vi "Time calculation.vi"(0 "Time between marks (ticks)":u32, 1 "Mode":enum16{"Auto Calc Tpulse", "Auto Calc Tb"}(ring), 5 "Ta (ticks)":i32, 7 "Tb (ticks)":i32, 9 "Number of pulses (N)":i32=4, 11 "TPulse (ticks)":i32=2000) -> (4 "appended array":i32[](array[numeric]), 6 "Ta Error":bool, 8 "Tb Error":bool, 10 "Tpulse Error":bool, 15 "Remainder (ticks)":i32)   [LabVIEW 2014]
panel:
  out "Tpulse OK?":bool
  out "Tb OK?":bool
  out "Ta OK?":bool
  out "Ta Out":i32
  out "Tb Out":i32
  out "TPulse Out":i32
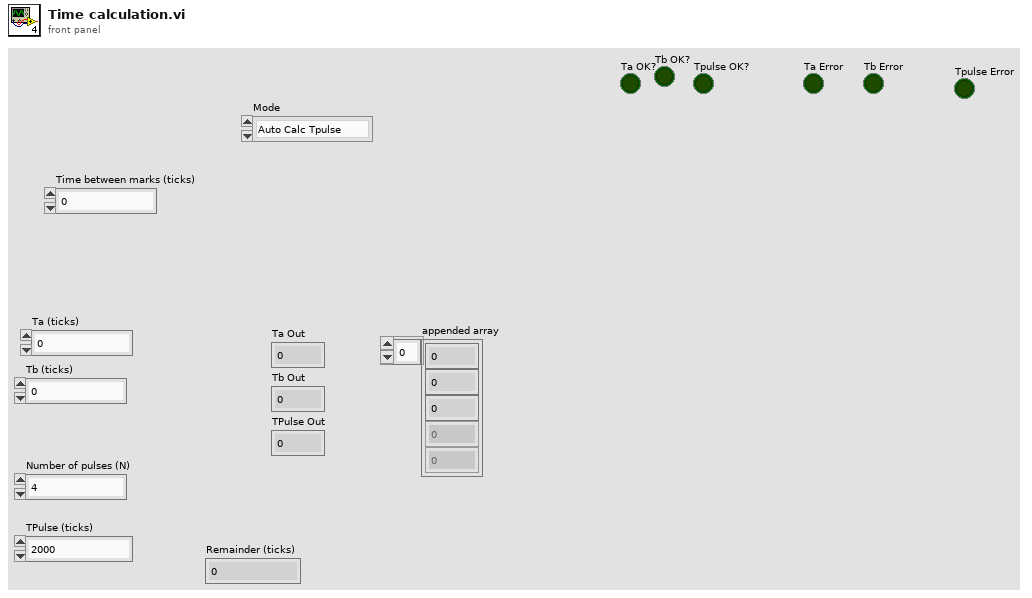
[diagram p1: front panel]
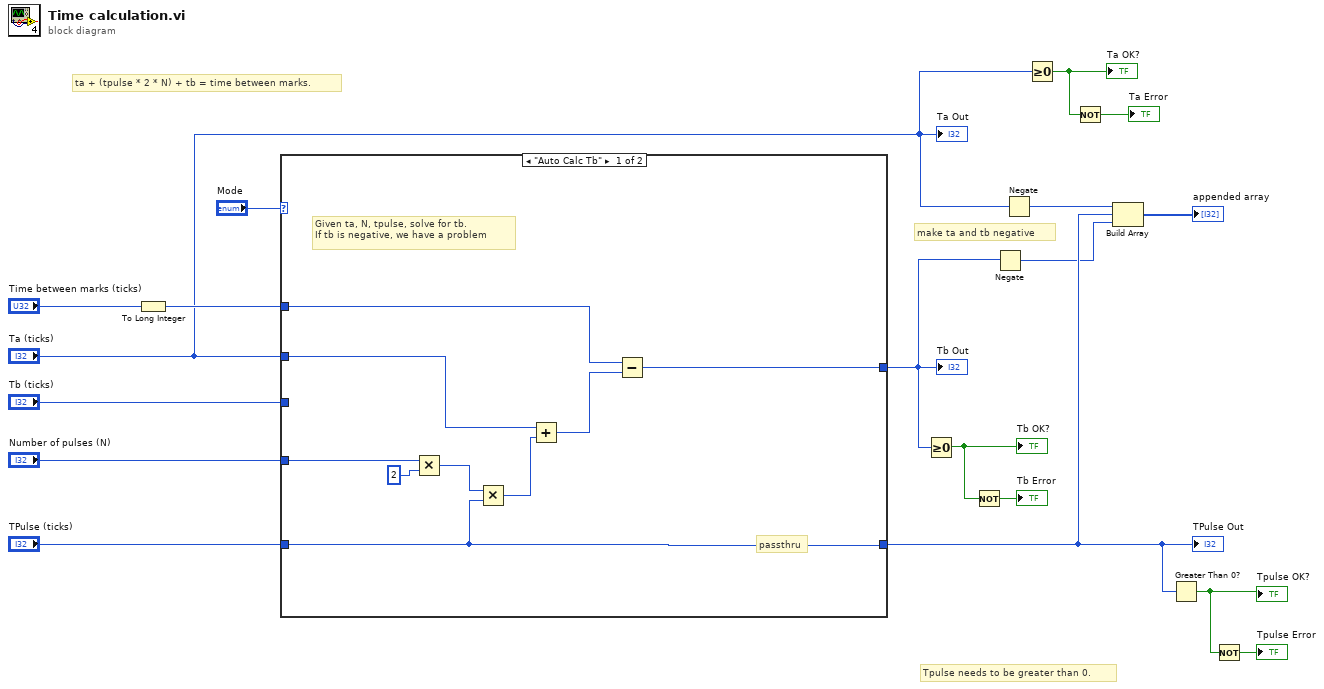
[diagram p0: block diagram]
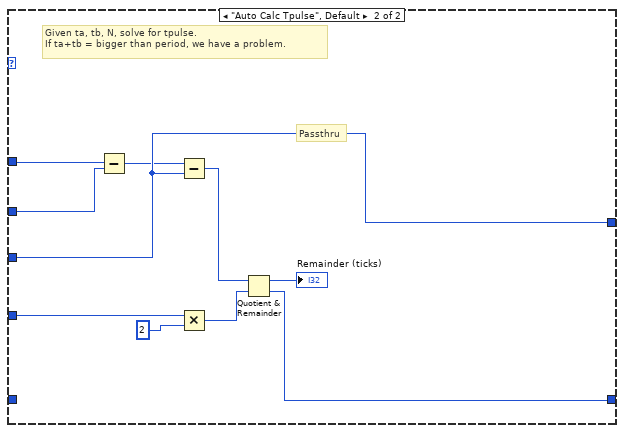
[diagram p2: hidden frame]
diagram:
  # "make ta and tb negative"
  # "Tpulse needs to be greater than 0."
  # "ta + (tpulse * 2 * N) + tb = time between marks."
  n1 = To Long Integer(number="Time between marks (ticks)") -> (32bit integer=w13:i32)
  n2 = case shown="\"Auto Calc Tb\"" "Mode" {
    tunnel: w13 -> [w21 w36]
    tunnel: "Ta (ticks)" -> [w23 w35]
    tunnel: "Tb (ticks)" -> [_ w34]
    tunnel: "Number of pulses (N)" -> [w26 w37]
    tunnel: "TPulse (ticks)" -> [w20 _]
    tunnel: [w20 w28] -> w12
    tunnel: [w19 w34] -> w5
    frame "Auto Calc Tb" {
      # "passthru"
      # "Given ta, N, tpulse, solve for tb.\nIf tb is negative, we have a problem"
      n3 = Multiply(x=w26, y=2) -> (x*y=w25:i32)
      n4 = Multiply(x=w25, y=w20) -> (x*y=w24:i32)
      n5 = Add(x=w23, y=w24) -> (x+y=w22:i32)
      n6 = Subtract(x=w21, y=w22) -> (x-y=w19:i32)
    }
    frame "Auto Calc Tpulse", Default {
      # "Passthru"
      # "Given ta, tb, N, solve for tpulse.\nIf ta+tb = bigger than period, we have a problem."
      n7 = Subtract(x=w36, y=w35) -> (x-y=w33:i32)
      n8 = Subtract(x=w33, y=w34) -> (x-y=w30:i32)
      n9 = Multiply(x=w37, y=2) -> (x*y=w31:i32)
      n10 = Quotient & Remainder(x=w30, y=w31) -> (x-y*floor(x/y)=→"Remainder (ticks)":i32, floor(x/y)=w28:i32)
    }
  }
  "TPulse Out" <- w12
  "Tb Out" <- w5
  n11 = Greater Or Equal To 0?(x=w5) -> (x >= 0?=w8:bool)
  "Tb OK?" <- w8
  n12 = Not(x=w8) -> (.not. x?=→"Tb Error":bool)
  n13 = Negate(x=w5) -> (-x=w4:i32)
  n14 = Negate(x="Ta (ticks)") -> (-x=w2:i32)
  n15 = Greater Or Equal To 0?(x="Ta (ticks)") -> (x >= 0?=w11:bool)
  "Ta OK?" <- w11
  n16 = Not(x=w11) -> (.not. x?=→"Ta Error":bool)
  n17 = Build Array(w2, w12, w4) -> (→"appended array":i32[])
  n18 = Greater Than 0?(x=w12) -> (x > 0?=w6:bool)
  "Tpulse OK?" <- w6
  n19 = Not(x=w6) -> (.not. x?=→"Tpulse Error":bool)
  "Ta Out" <- "Ta (ticks)"
